vi "Real Schur Decomposition.vi"(9 "order":T1 items=["No Reorder", "Real Ascending", "Real Descending", "Magnitude Ascending", "Magnitude Descending"], 10 "compute Schur vectors?":bool, 11 "Input Matrix":T2) -> (0 "error":i32, 1 "Eigenvalues":cdb[](array[numeric]), 2 "Schur Vectors":T2, 3 "Schur Form":T2)   [LabVIEW 2020, in "NI_AALPro.lvlib"]
doc: "Performs the Schur decomposition of a square matrix. Wire data to the <B>Input Matrix</B> input to determine the polymorphic instance to use or manually select the instance."
uses:
  <vilib>/Analysis/NI_AALPro.lvlib
  <vilib>/Analysis/Matrix/Datatypes/RealMatrix.ctl
  <vilib>/Analysis/7linalg.llb/Eigenvalue Order.ctl
  <resource>/lvanlys.dll
  <vilib>/Analysis/Matrix/NI_Matrix.lvlib
panel:
  # "Schur Decomposition"
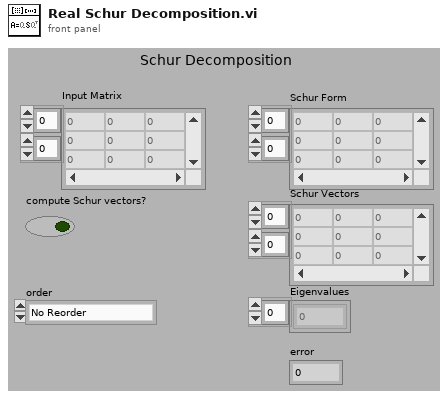
[diagram p1: front panel]
types:
  T1 = typedef "NI_AALPro.lvlib/Eigenvalue Order.ctl" = u16
  T2 = typedef "NI_Matrix.lvlib/RealMatrix.ctl" = dbl[][]
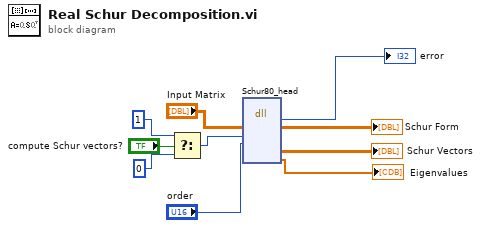
[diagram p0: block diagram]
diagram:
  n1 = Select(t=1, s="compute Schur vectors?", f=0) -> (s? t:f=w7:i32)
  n2 = dll-call lib="e:/builds/penguin/labview/branches/2020/dev/dist/resource/lvanlys.*" fn="Schur80_head"("Input Matrix"="Input Matrix", "compSV"=w7, "orderOpt"="order") -> (→"error":i32, "Input Matrix"=→"Schur Form":T2, "Schur Vectors"=→"Schur Vectors":T2, "Eigenvalues"=→"Eigenvalues":cdb[])  [unwired: 7 in, 2 out]
